vi "Write task.vi"(8 "error in (no error)":errorcluster, 10 "task":refnum<k21>, 11 "NI_DAQmx(AI) in":refnum<class "NI_DAQmx(AI).lvclass">) -> (0 "error out":errorcluster, 3 "NI_DAQmx(AI) out":refnum<class "NI_DAQmx(AI).lvclass">)   [LabVIEW 2025, in "NI_DAQmx(AI).lvclass"]
uses:
  NI_DAQmx(AI).lvclass
  NI_DAQmx(AI).lvclass/NI_DAQmx(AI).ctl
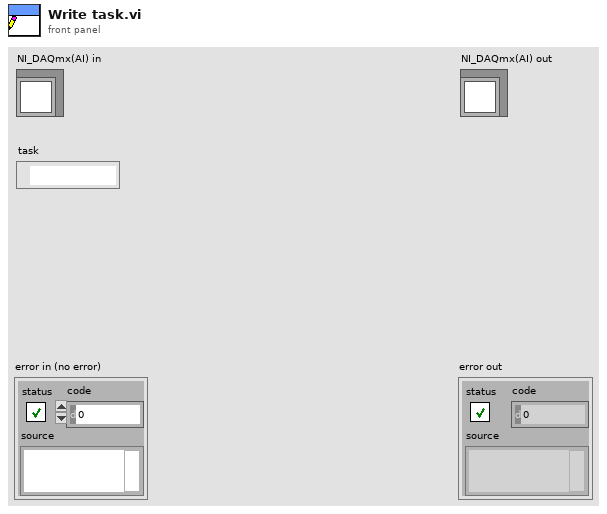
[diagram p1: front panel]
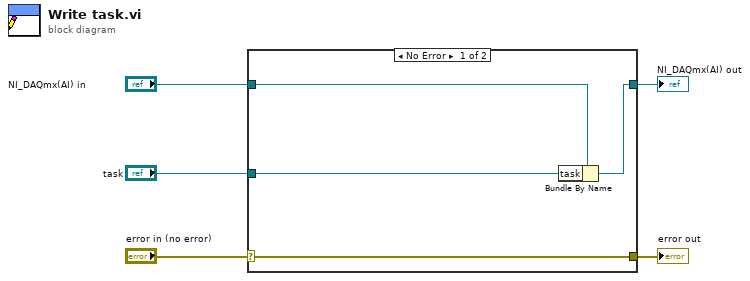
[diagram p0: block diagram]
diagram:
  n1 = case shown="No Error" "error in (no error)" {
    selector: "error in (no error)" -> [w9 w10]
    tunnel: [w9 w10] -> w4
    tunnel: [w7 w11] -> w2
    tunnel: "NI_DAQmx(AI) in" -> [w8 w11]
    tunnel: "task" -> [w6 _]
    frame No Error {
      n2 = Bundle By Name(cluster=w8, "task"=w6) -> (w7:refnum<class "NI_DAQmx(AI).lvclass">)
    }
    frame Error {
    }
  }
  "error out" <- w4
  "NI_DAQmx(AI) out" <- w2
